vi "Read Remaining Output.vi"(8 "error in (no error)":errorcluster, 11 "connection in":refnum<class "Low Level Connection.lvclass">) -> (0 "error out":errorcluster, 3 "connection out":refnum<class "Low Level Connection.lvclass">)   [LabVIEW 2020, in "NI_SFTP.lvlib" / "Low Level Connection.lvclass"]
uses:
  <vilib>/net/SFTP/Low Level Connection/Low Level Connection.lvclass
  <vilib>/Utility/Deadline/Mode.ctl
  <vilib>/Utility/Deadline/NI_Deadline.lvlib
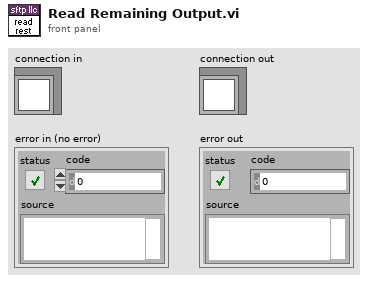
[diagram p1: front panel]
types:
  T1 = typedef "NI_Deadline.lvlib/Mode.ctl" = enum16{"Relative", "Use deadline", "Wait forever", "Nonblocking", "N/A"}
  T2 = typedef "NI_Deadline.lvlib/Deadline.ctl" = cluster{"mode":T1, "deadline (ms)":u32}
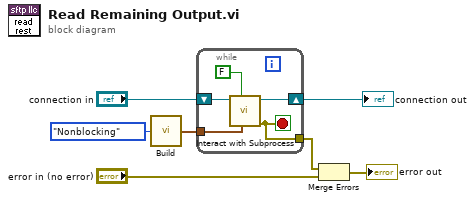
[diagram p0: block diagram]
diagram:
  n1 = call <vilib>:"Build.vi"("mode"=Mode."Nonblocking") -> ("Deadline out"=w4:T2)  [unwired: 2 in]
  n2 = while {
    shift-right: [w11] -> w2
    shift-left: "connection in" -> [w12]
    tunnel: [w10] -> w1
    tunnel: w4 -> [w8]
    stop <- w10 stop-if-true
    n3 = call <vilib>:"Interact with Subprocess.vi"("deadline"=w8, "check id"=FALSE ("check id?"), "connection in"=w12) -> ("error out"=w10:errorcluster, "connection out"=w11:refnum<class "Low Level Connection.lvclass">)  [unwired: 7 in]
  }
  "connection out" <- w2
  n4 = Merge Errors(w1, "error in (no error)") -> (→"error out":errorcluster)
